vi "Motion_Read Positions.vi"(8 "error in":errorcluster, 11 "TCP Connection Refnum in":refnum<k5>) -> (0 "error out":errorcluster, 1 "Loader Position":dbl format="%#_8g", 2 "Gantry Position":T1, 3 "TCP Connection Refnum (dup)":refnum<k5>, 4 "Exception Code":u8 format="%.0x", 5 "Raw Registers":u16[](array[numeric]))   [LabVIEW 2010]
uses:
  <vilib>/NI Modbus.llb/MB Ethernet Master Query Read Input Registers (poly).vi
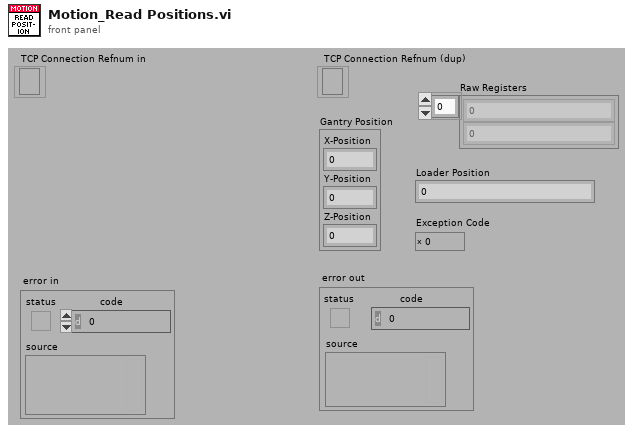
[diagram p1: front panel]
types:
  T1 = cluster{"X-Position":dbl, "Y-Position":dbl, "Z-Position":dbl}
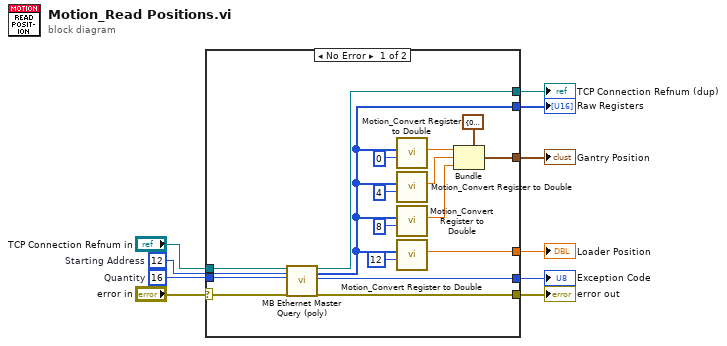
[diagram p0: block diagram]
diagram:
  w9 = u16 16  # Quantity
  w10 = u16 12  # Starting Address
  n1 = case shown="No Error" "error in" {
    selector: "error in" -> [w11 w30]
    tunnel: w10 -> [w28 _]
    tunnel: w9 -> [w27 _]
    tunnel: [w26 _] -> w8
    tunnel: [w21 _] -> w7
    tunnel: [w20 _] -> w6
    tunnel: "TCP Connection Refnum in" -> [w19 w29]
    tunnel: [w18 w30] -> w4
    tunnel: [w17 w29] -> w3
    tunnel: [w12 _] -> w2
    frame No Error {
      n2 = call-poly <vilib>:"MB Ethernet Master Query (poly).vi"("TCP Connection Refnum in"=w19, "Starting Address"=w28, "Quantity"=w27, "error in"=w11) -> ("TCP Connection Refnum (dup)"=w17:refnum<k5>, "Input Registers"=w20:u16[], "Exception Code"=w26:u8, "error out"=w18:errorcluster)  [unwired: 12 in]
      n3 = call "Motion_Convert Register to Double.vi"("Start index"=0, "Register array"=w20) -> ("Double Value"=w16:dbl)  [unwired: 7 in]
      n4 = call "Motion_Convert Register to Double.vi"("Start index"=4, "Register array"=w20) -> ("Double Value"=w15:dbl)  [unwired: 7 in]
      n5 = call "Motion_Convert Register to Double.vi"("Start index"=8, "Register array"=w20) -> ("Double Value"=w14:dbl)  [unwired: 7 in]
      n6 = call "Motion_Convert Register to Double.vi"("Start index"=12, "Register array"=w20) -> ("Double Value"=w21:dbl)  [unwired: 7 in]
      n7 = Bundle(cluster=T1 {"X-Position"=0.0, "Y-Position"=0.0, "Z-Position"=0.0}, "X-Position"=w16, "Y-Position"=w15, "Z-Position"=w14) -> (w12:T1)
    }
    frame Error {
    }
  }
  "Raw Registers" <- w6
  "Exception Code" <- w8
  "Loader Position" <- w7
  "error out" <- w4
  "TCP Connection Refnum (dup)" <- w3
  "Gantry Position" <- w2
